vi "generateSetpoints.vi"(11 "Motion profile":cluster{"time (s)":dbl, "velocity":dbl}[](array[cluster])) -> (2 "profile complete?":bool, 3 "Setpoints":cluster{"accel":dbl, "vel":dbl, "pos":dbl})   [LabVIEW 2015]
uses:
  <vilib>/addons/control/pid/NI_PID_pid.lvlib
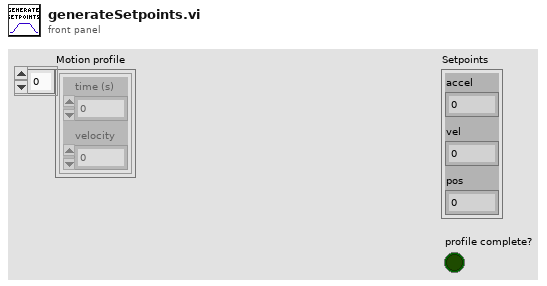
[diagram p1: front panel]
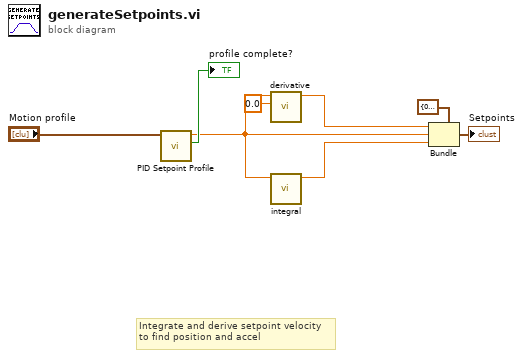
[diagram p0: block diagram]
diagram:
  # "Integrate and derive setpoint velocity\nto find position and accel"
  n1 = call <vilib>:"PID Setpoint Profile.vi"("setpoint profile"="Motion profile") -> ("profile complete?"=→"profile complete?":bool, "setpoint"=w3:dbl)  [unwired: 5 in, 2 out]
  n2 = call "derivative.vi"("Starting value"=0.0, "x"=w3) -> ("dx/dt"=w4:dbl)  [unwired: 9 in]
  n3 = call "integral.vi"("x"=w3) -> ("Integral x"=w2:dbl)  [unwired: 10 in]
  n4 = Bundle(cluster=cluster{"accel":dbl, "vel":dbl, "pos":dbl} {"accel"=0.0, "vel"=0.0, "pos"=0.0}, "accel"=w4, "vel"=w3, "pos"=w2) -> (→"Setpoints":cluster{"accel":dbl, "vel":dbl, "pos":dbl})
